vi "resistor initial.vi"(8 "error in":errorcluster caption="에러 입력", 10 "Sample Number":i32=100, 11 "Sampling rate":dbl=1000.0) -> (0 "error out":errorcluster caption="에러 출력", 3 "task out":refnum<k21> caption="태스크 출력")   [LabVIEW 2013]
uses:
  <vilib>/DAQmx/configure/timing.llb/DAQmx Timing (Sample Clock).vi
  <vilib>/DAQmx/create/channels.llb/DAQmx Create Channel (AI-Voltage-Basic).vi
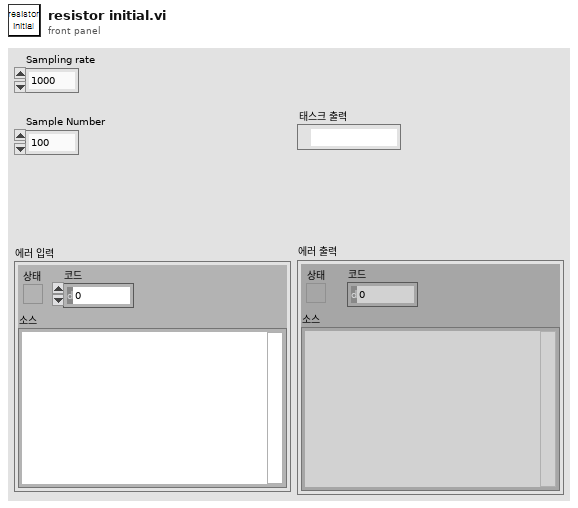
[diagram p1: front panel]
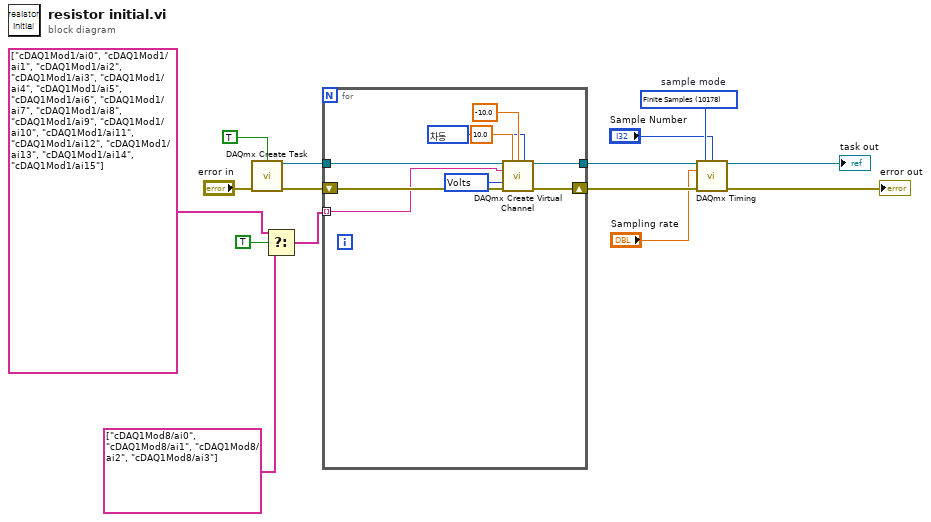
[diagram p0: block diagram]
diagram:
  w10 = 10178 items=["Finite Samples"=10178, "Continuous Samples"=10123, "Hardware Timed Single Point"=12522]  # sample mode
  n1 = call <vilib>:"DAQmx Create Task.vi"("auto cleanup"=TRUE, "error in"="error in") -> ("task out"=w13:refnum<k21>, "error out"=w15:errorcluster)  [unwired: 12 in]
  n2 = Select(t=tag[] ["cDAQ1Mod1/ai0", "cDAQ1Mod1/ai1", "cDAQ1Mod1/ai2", "cDAQ1Mod1/ai3", "cDAQ1Mod1/ai4", "cDAQ1Mod1/ai5", "cDAQ1Mod1/ai6", "cDAQ1Mod1/ai7", "cDAQ1Mod1/ai8", "cDAQ1Mod1/ai9", "cDAQ1Mod1/ai10", "cDAQ1Mod1/ai11", "cDAQ1Mod1/ai12", "cDAQ1Mod1/ai13", "cDAQ1Mod1/ai14", "cDAQ1Mod1/ai15"], s=TRUE, f=tag[] ["cDAQ1Mod8/ai0", "cDAQ1Mod8/ai1", "cDAQ1Mod8/ai2", "cDAQ1Mod8/ai3"]) -> (s? t:f=w6:tag[])
  n3 = for "For 루프" {
    tunnel: w13 -> [w24]
    tunnel: [w22] -> w11
    shift-right: [w21] -> w12
    shift-left: w15 -> [w23]
    tunnel: w6 -> [w16] mode=indexing
    w17 = 10348 items=["Volts"=10348, "사용자 스케일로부터"=10065] ("units")
    w18 = 10106 items=["기본값"=-1, "RSE"=10083, "NRSE"=10078, "차동"=10106, "유사 차동"=12529] ("input terminal configuration")
    n4 = call-poly <vilib>:"DAQmx Create Virtual Channel.vi"("task in"=w24, "maximum value"=10.0, "minimum value"=-10.0, "input terminal configuration"=w18, "physical channels"=w16, "units"=w17, "error in"=w23) -> ("task out"=w22:refnum<k21>, "error out"=w21:errorcluster)  [unwired: 7 in]
  }
  n5 = call-poly <vilib>:"DAQmx Timing.vi"("task/channels in"=w11, "sample mode"=w10, "samples per channel"="Sample Number", "rate"="Sampling rate", "error in"=w12) -> ("task out"=→"task out":refnum<k21>, "error out"=→"error out":errorcluster)  [unwired: 9 in]
